vi "Feedback [R]s.vi"(2 "L/R":bool, 3 "Marker 2":dbl[](array[numeric]), 4 "Origin":dbl[](array[numeric]), 5 "Marker 1":dbl[](array[numeric])) -> (0 "[R]T":dbl[][](array[numeric]), 1 "[R]":dbl[][](array[numeric]))   [LabVIEW 2010]
uses:
  <vilib>/Analysis/baseanly.llb/Unit Vector (DBL).vi
  <vilib>/Analysis/NI_AALBase.lvlib
  <vilib>/Analysis/NI_AALPro.lvlib
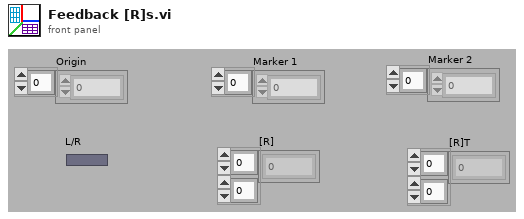
[diagram p1: front panel]
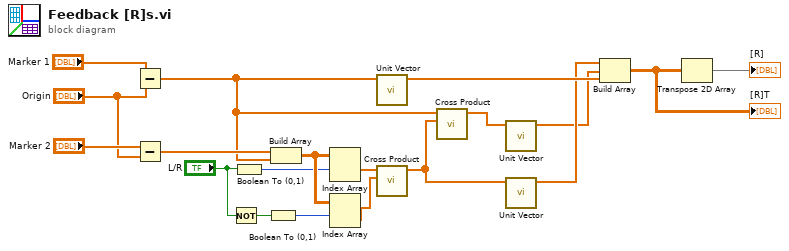
[diagram p0: block diagram]
diagram:
  n1 = Subtract(x="Marker 1", y="Origin") -> (x-y=w2:dbl[])
  n2 = Subtract(x="Marker 2", y="Origin") -> (x-y=w10:dbl[])
  n3 = Not(x="L/R") -> (.not. x?=w7:bool)
  n4 = Boolean To (0,1)(Boolean="L/R") -> (0, 1=w5:i16)
  n5 = Boolean To (0,1)(Boolean=w7) -> (0, 1=w6:i16)
  n6 = Build Array(w10, w2) -> (w9:dbl[][])
  n7 = Index Array(array=w9, index (row)=w5) -> (element=w4:dbl[])  [unwired: 1 in]
  n8 = Index Array(array=w9, index (row)=w6) -> (element=w3:dbl[])  [unwired: 1 in]
  n9 = call-poly <vilib>:"Unit Vector.vi"("Input Vector"=w2) -> ("Unit Vector"=w16:dbl[])  [unwired: 8 in, 2 out]
  n10 = call <vilib>:"Cross Product.vi"("B Vector"=w3, "A Vector"=w4) -> ("Cross Product"=w1:dbl[])  [unwired: 8 in, 1 out]
  n11 = call <vilib>:"Cross Product.vi"("B Vector"=w1, "A Vector"=w2) -> ("Cross Product"=w17:dbl[])  [unwired: 8 in, 1 out]
  n12 = call-poly <vilib>:"Unit Vector.vi"("Input Vector"=w17) -> ("Unit Vector"=w14:dbl[])  [unwired: 8 in, 2 out]
  n13 = call-poly <vilib>:"Unit Vector.vi"("Input Vector"=w1) -> ("Unit Vector"=w15:dbl[])  [unwired: 8 in, 2 out]
  n14 = Build Array(w15, w14, w16) -> (w19:dbl[][])
  "[R]T" <- w19
  n15 = Transpose 2D Array(2D array=w19) -> (transposed array=→"[R]":dbl[][])
